vi "Kinesis - KDC101 - No Front Panel.vi"() -> ()   [LabVIEW 2021]
uses:
  C:/Users/arjun/Documents/Spring 22/Edited_PMT_code_for_upload/Data_Acq_test/SampleCodeLabView/Kinesis_with_LabVIEW_Examples_LV12 - v3/Thorlabs.MotionControl.DeviceManagerCLI.dll
  Thorlabs.MotionControl.DeviceManagerCLI.dll
  C:/Users/arjun/Documents/Spring 22/Edited_PMT_code_for_upload/Data_Acq_test/SampleCodeLabView/Kinesis_with_LabVIEW_Examples_LV12 - v3/ThorLabs.MotionControl.KCube.DCServoCLI.dll
  ThorLabs.MotionControl.KCube.DCServoCLI.dll
  C:/Users/arjun/Documents/Spring 22/Edited_PMT_code_for_upload/Data_Acq_test/SampleCodeLabView/Kinesis_with_LabVIEW_Examples_LV12 - v3/Thorlabs.MotionControl.GenericMotorCLI.dll
  Thorlabs.MotionControl.GenericMotorCLI.dll
panel:
  out "Moving":bool
  out "Controller Information":T1
  in  "Type the name of the Stage/Actuator e.g. MTS50/M-Z8":string
  in  "serialNo":string
  # "Thorlabs Hardware: KDC101 - K-Cube Brushed DC Servo Motor Controller\n https://www.thorlabs.com/thorproduct.cfm?partnumber=KDC101\n\nDescription: This VI is an example of communicating with Thorlabs Motion Control devices outside of the provided WinForms UI controls contained in Thorlabs.MotionControl.Controls.dll.\nInstead, we introduce how you can make use of the wider range of Generic & Device-specific component DLLs included with your Kinesis Installation. \n\nThe VI will identify & connect to your KDC101 through BuildDeviceList() & assign Motor Settings based on the actuator/stage name entered into the control detailed in the ThorlabsDefaultSettings file. \nDevice information will output to the 'Controller Information' cluster & then he connected device will perform a 'Home'. A Virtual Boolean LED will identify whether the device is moving & will end the program when the device is 'Homed'.\n\nInstructions: \n1) Connect your KDC101 device to your PC & power the device, ensuring your stage/actutator is connected. For full device setup, \nthe device product manual can be found on our website here. - https://www.thorlabs.com/thorproduct.cfm?partnumber=KDC101\n2) Enter the device serial number & actuator/stage name to the left. To ensure the correct string is used, you can copy your Stage/Actuator Part Number from ThorlabsDefaultSettings file found in: \nC:\\Program Files (x86)\\Thorlabs\\Kinesis or\nC:\\Program Files\\Thorlabs\\Kinesis\n\n3) Click 'Run' in the LabVIEW Toolbar."
  # "Notes:"
  # "- Open the example VI through the LabVIEW Project Explorer to correctly load the dlls.\n\n\n\n\n\n\n\n\n\n\n\n\n- To explore the range of methods available, please visit the .NET API, included with your Kinesis software.\n\n- For tips on building your own VIs with Thorlabs Motion Control Hardware, please see our LabVIEW Guide here.\nhttps://www.thorlabs.com/newgrouppage9.cfm?objectgroup_id=10285"
  # "- Ensure that the appropriate .DLLs are copied into your Project Folder. Check that the correct bit type are used depending on your version of LabVIEW\ni.e. 32-bit or 64-bit."
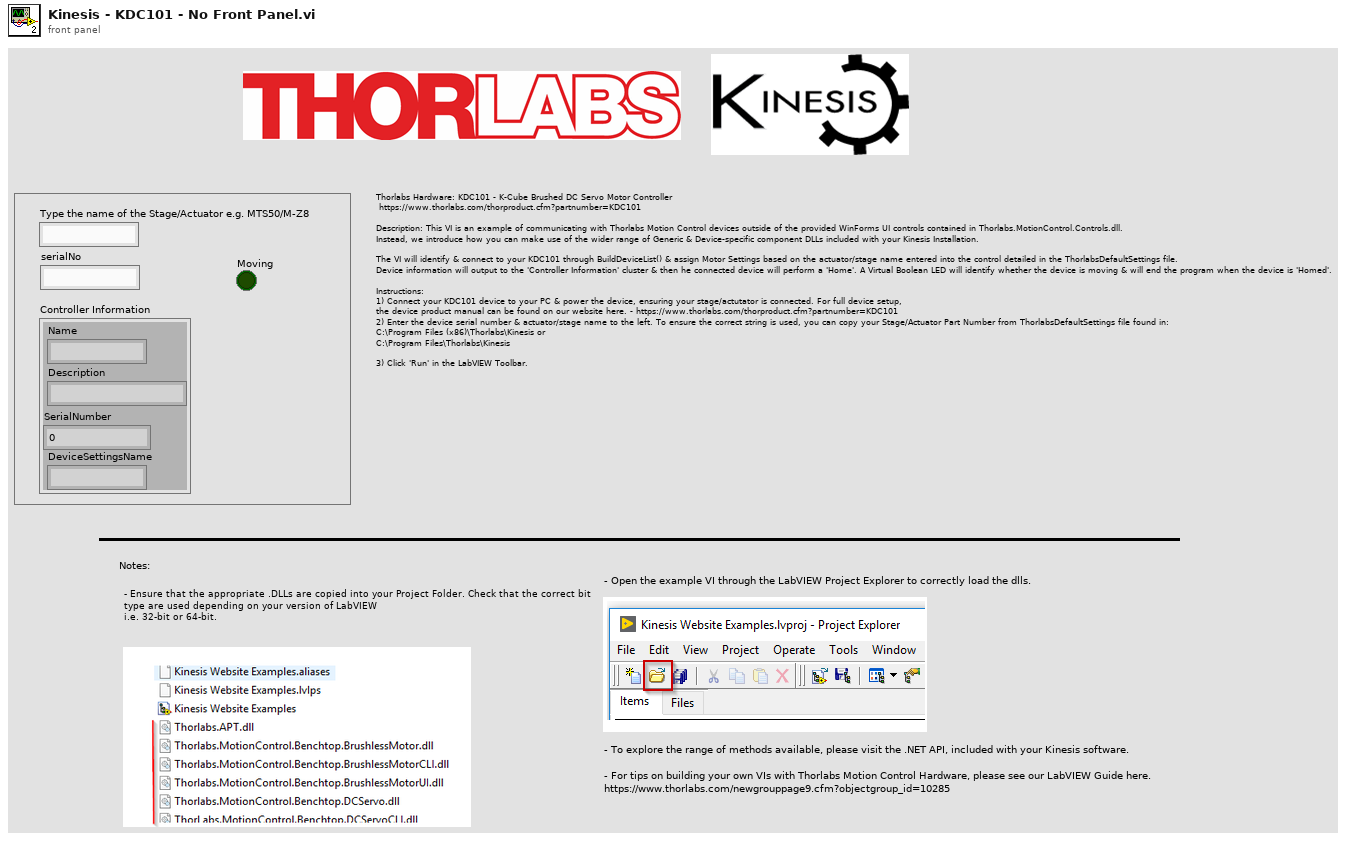
[diagram p1: front panel]
types:
  T1 = cluster{"Name":string, "Description":string, "SerialNumber":u32, "DeviceSettingsName":string}
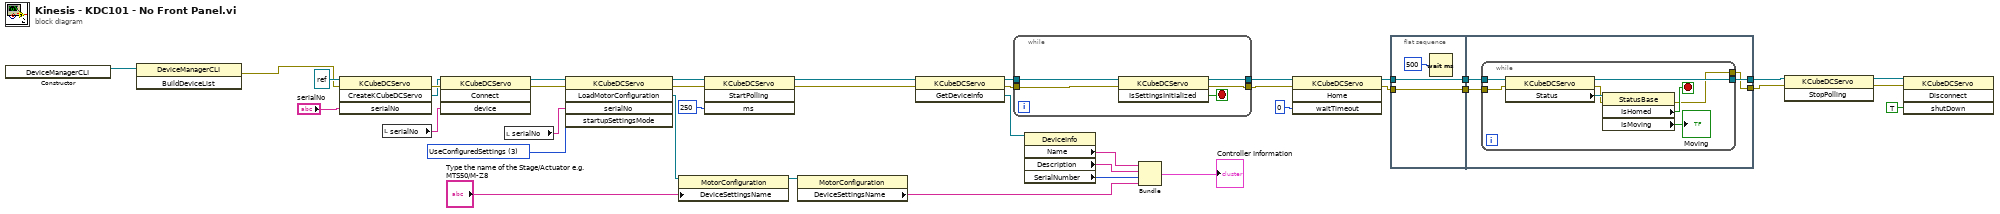
[diagram p0: block diagram]
diagram:
  w18 = 3 items=["UseDeviceSettings"=1, "UseFileSettings"=2, "UseConfiguredSettings"=3] ("startupSettingsMode")
  n1 = constructor class="DeviceManagerCLI"() -> (reference out=w7:refnum<k24>)  [unwired: 3 in, 2 out]
  n2 = invoke class="DeviceManagerCLI" method="BuildDeviceList"(reference=w7) -> (error out=w6:errorcluster)  [unwired: 2 in, 2 out]
  n3 = invoke class="KCubeDCServo" method="CreateKCubeDCServo"(reference=refnum<k24> refnum ("target class"), error in=w6, "serialNo"="serialNo") -> (error out=w38:errorcluster, "CreateKCubeDCServo"=w35:refnum<k24>)  [unwired: 1 in, 2 out]
  n4 = local read "serialNo"() -> (w37:string)
  n5 = invoke class="KCubeDCServo" method="Connect"(reference=w35, error in=w38, "device"=w37) -> (reference out=w16:refnum<k24>, error out=w14:errorcluster)  [unwired: 1 in, 2 out]
  n6 = local read "serialNo"() -> (w15:string)
  n7 = invoke class="KCubeDCServo" method="LoadMotorConfiguration"(reference=w16, error in=w14, "serialNo"=w15, "startupSettingsMode"=w18) -> (reference out=w33:refnum<k24>, error out=w13:errorcluster, "LoadMotorConfiguration"=w26:refnum<k24>)  [unwired: 1 in, 2 out]
  n8 = property class="MotorConfiguration"(reference=w26, "DeviceSettingsName"="Type the name of the Stage/Actuator e.g. MTS50/M-Z8") -> (reference out=w29:refnum<k24>)  [unwired: 1 in, 1 out]
  n9 = invoke class="KCubeDCServo" method="StartPolling"(reference=w33, error in=w13, "ms"=250) -> (reference out=w28:refnum<k24>, error out=w12:errorcluster)  [unwired: 1 in, 2 out]
  n10 = property class="MotorConfiguration"(reference=w29) -> ("DeviceSettingsName"=w30:string)  [unwired: 1 in, 2 out]
  n11 = invoke class="KCubeDCServo" method="GetDeviceInfo"(reference=w28, error in=w12) -> (reference out=w22:refnum<k24>, error out=w11:errorcluster, "GetDeviceInfo"=w21:refnum<k24>)  [unwired: 1 in]
  n12 = while {
    tunnel: [w43] -> w20
    tunnel: w22 -> [w44]
    tunnel: w11 -> [w41]
    tunnel: [w40] -> w10
    stop <- w42 stop-if-true
    n13 = invoke class="KCubeDCServo" method="IsSettingsInitialized"(reference=w44, error in=w41) -> (reference out=w43:refnum<k24>, error out=w40:errorcluster, "IsSettingsInitialized"=w42:bool)  [unwired: 1 in]
  }
  n14 = property class="DeviceInfo"(reference=w21) -> ("Name"=w23:string, "Description"=w24:string, "SerialNumber"=w25:u32)  [unwired: 1 in, 2 out]
  n15 = Bundle("Name"=w23, "Description"=w24, "SerialNumber"=w25, "DeviceSettingsName"=w30) -> (→"Controller Information":T1)  [unwired: 1 in]
  n16 = invoke class="KCubeDCServo" method="Home"(reference=w20, error in=w10, "waitTimeout"=0) -> (reference out=w32:refnum<k24>, error out=w8:errorcluster)  [unwired: 1 in, 2 out]
  n17 = flat-sequence {
    tunnel: [w46] -> w34
    tunnel: w32 -> [w46]
    tunnel: [w45] -> w9
    tunnel: w8 -> [w45]
    tunnel: [w51] -> w5
    tunnel: w34 -> [w50]
    tunnel: w9 -> [w49]
    tunnel: [w48] -> w4
    frame #0 {
      n18 = Wait (ms)(milliseconds to wait=u32 500) -> ()  [unwired: 1 out]
    }
    frame #1 {
      n19 = while {
        tunnel: [w56] -> w51
        tunnel: w50 -> [w57]
        tunnel: w49 -> [w54]
        tunnel: [w52] -> w48
        stop <- w55 stop-if-true
        n20 = property class="KCubeDCServo"(reference=w57, error in=w54) -> (reference out=w56:refnum<k24>, error out=w53:errorcluster, "Status"=w58:refnum<k24>)
        n21 = property class="StatusBase"(reference=w58, error in=w53) -> (error out=w52:errorcluster, "IsHomed"=w55:bool, "IsMoving"=→"Moving":bool)  [unwired: 1 out]
      }
    }
  }
  n22 = invoke class="KCubeDCServo" method="StopPolling"(reference=w5, error in=w4) -> (reference out=w3:refnum<k24>, error out=w2:errorcluster)  [unwired: 1 in, 1 out]
  n23 = invoke class="KCubeDCServo" method="Disconnect"(reference=w3, error in=w2, "shutDown"=TRUE) -> ()  [unwired: 1 in, 4 out]
